vi "bmp_2_mat.vi"(9 "Destinatia1":path, 11 "Imaginea1":path) -> ()   [LabVIEW 2015]
uses:
  <vilib>/picture/picture.llb/Draw True-Color Pixmap.vi
panel:
  out "new":u8[][](array[numeric]) format="%x"
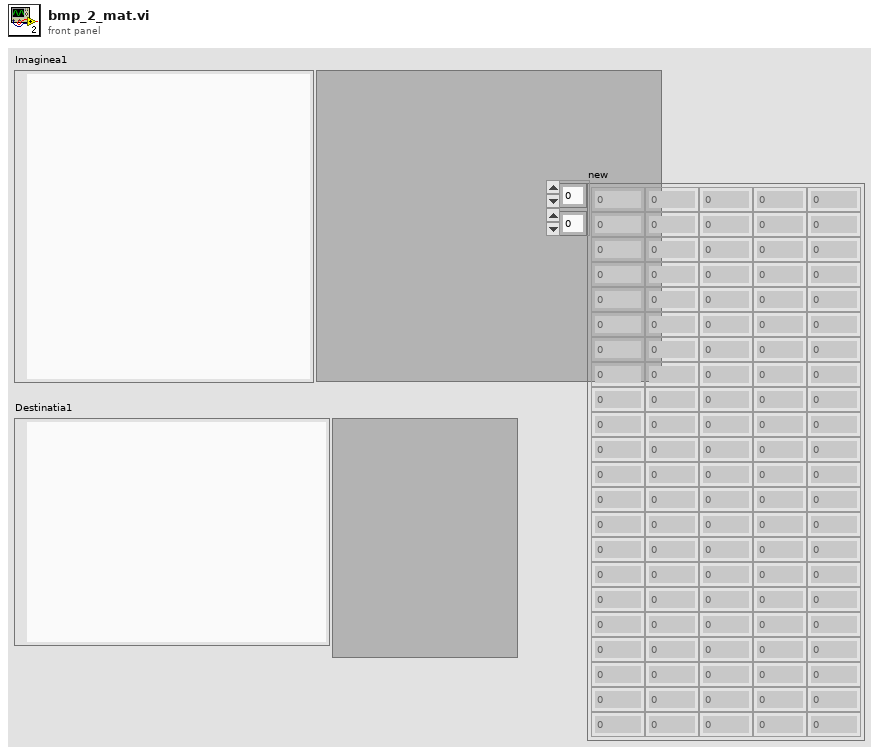
[diagram p1: front panel]
types:
  T1 = typedef "imagedata.ctl" = cluster{"image type":i32, "image depth":i32, "image":u8[], "mask":u8[], "colors":u32[], "Rectangle":cluster{"left":i16, "top":i16, "right":i16, "bottom":i16}}
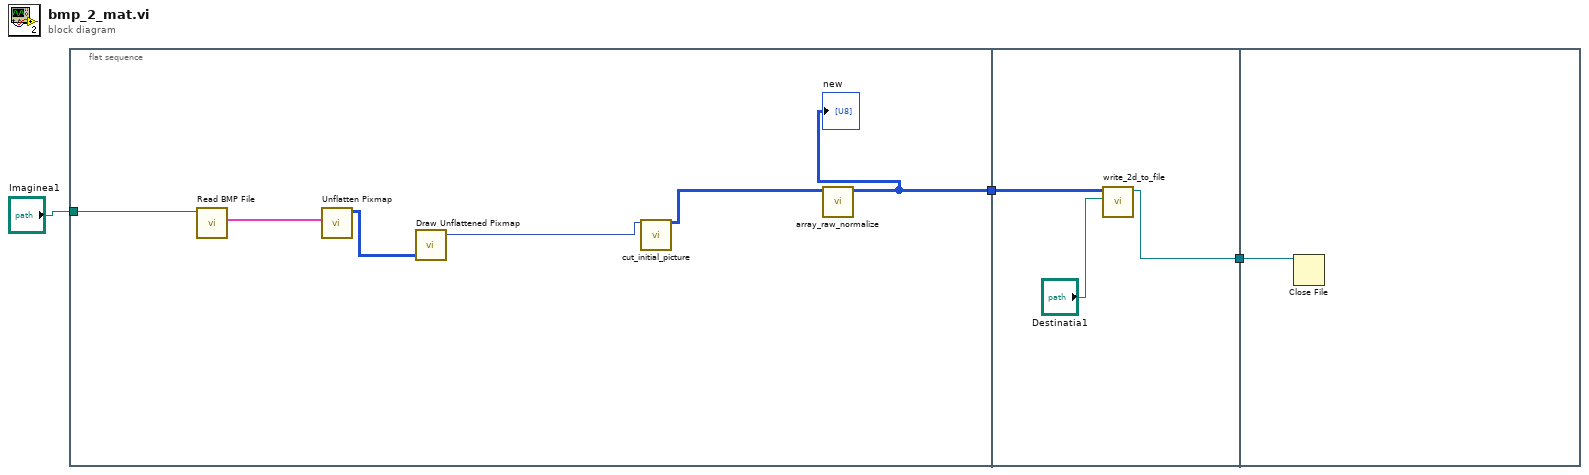
[diagram p0: block diagram]
diagram:
  n1 = flat-sequence {
    tunnel: [w4] -> w3
    tunnel: "Imaginea1" -> [w8]
    tunnel: w3 -> [w12]
    tunnel: [w10] -> w2
    tunnel: w2 -> [w13]
    frame #0 {
      n2 = call <vilib>:"Read BMP File.vi"("path to BMP file"=w8) -> ("image data"=w9:T1)  [unwired: 8 in, 2 out]
      n3 = call <vilib>:"Unflatten Pixmap.vi"("image data"=w9) -> ("24-bit pixmap"=w7:u32[][])  [unwired: 4 in, 6 out]
      n4 = call-poly <vilib>:"Draw Unflattened Pixmap.vi"("data (RGB format)"=w7) -> ("new picture"=w6:picture)  [unwired: 8 in]
      n5 = call "cut_initial_picture.vi"("picture"=w6) -> ("new"=w5:u32[][])  [unwired: 14 in]
      n6 = call "array_raw_normalize.vi"("array"=w5) -> ("Array"=w4:u8[][])  [unwired: 10 in]
      "new" <- w4
    }
    frame #1 {
      n7 = call "write_2d_to_file.vi"("Path 2"="Destinatia1", "Array"=w12) -> ("refnum out"=w10:refnum<file>)  [unwired: 9 in]
    }
    frame #2 {
      n8 = Close File(refnum=w13) -> ()  [unwired: 1 in, 2 out]
    }
  }
